vi "FTW-Package-Lossy-CreateQueue.vi"(9 "max queue size (1)":i32=1, 11 "error in":errorcluster) -> (4 "Queue":refnum<queue>, 15 "error out":errorcluster)   [LabVIEW 2013, in "FTW-Package-Lossy.lvclass"]
uses:
  FTW-Package-Lossy.lvclass
  Message/FTW-Message.ctl
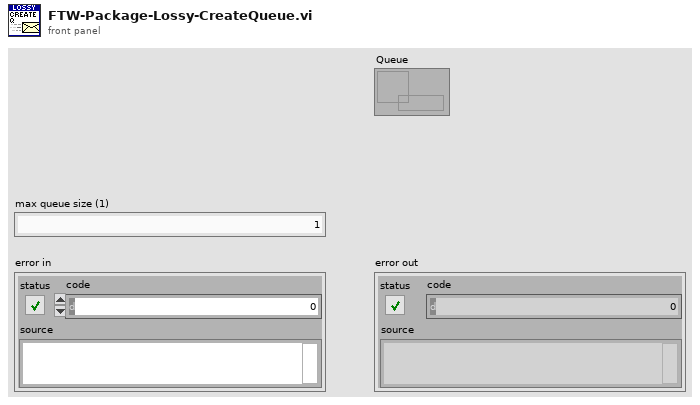
[diagram p1: front panel]
types:
  T1 = typedef "FTW-Message.ctl" = cluster{"Header":string, "Body":string, "Metadata":string}
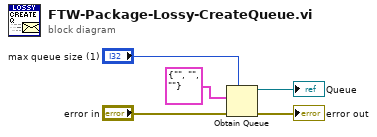
[diagram p0: block diagram]
diagram:
  n1 = Obtain Queue(max queue size (-1, unlimited)="max queue size (1)", element data type=T1 {"Header"="", "Body"="", "Metadata"=""} ("Parts"), error in (no error)="error in") -> (queue out=→"Queue":refnum<queue>, error out=→"error out":errorcluster)  [unwired: 2 in, 1 out]
